vi "Stoppani File Read.vi"(0 "String in":path) -> (3 "run":cluster{"Sampling rate":dbl, "npts":dbl}, 4 "Waveform Graph":T1(graph), 5 "Header Info":T2={"TFRFHeader"={"index"=22, "Xr"=294.1319931548027, "Yr"=349.0, "XActual"=294.1319931548027, "YActual"=349.0}, "Frequency Axis"={"Hz Resolution"=0.67291259765625, "Start Freq"=24.89776611328125, "End Freq"=3500.4913330078125}, "TSingleArray"={"fComplex"=1, "fLength"=5166.0, "a[2]"=0.0, "fConditionCheck"=1.0, "Precision"=0.0, "MtxVecVersion"=420.0, "SizeOf(TSample)"=8.0, "Tag"=0.0, "MtxVecFileCode"=64019.0, "a[9]"=0.0, "a[10]"=0.0}, "caption"="\u0000\u0000\u0000\u0000"}, 6 "Complex FRF":cluster{"t0":dbl, "dt":dbl, "Y":cdb[]})   [LabVIEW 2022 SP3]
panel:
  out "String out":string
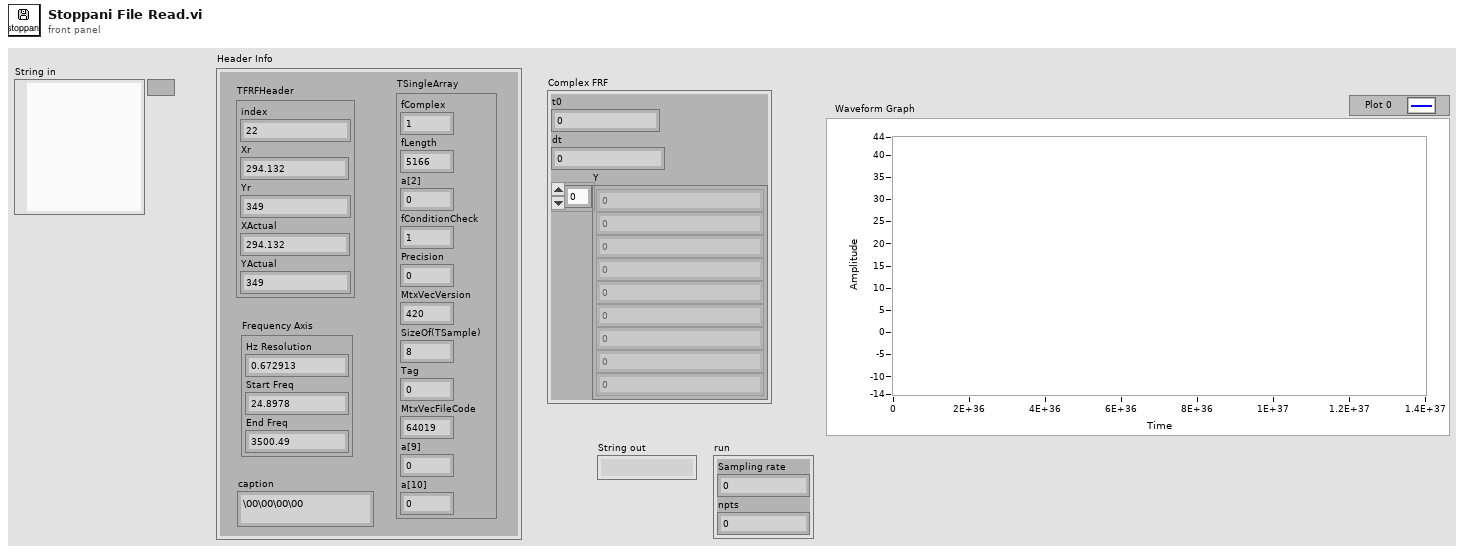
[diagram p1: front panel]
types:
  T1 = cluster{"Start freq":dbl, "Hz resolution":dbl, dbl[]}
  T2 = cluster{"TFRFHeader":cluster{"index":u32, "Xr":dbl, "Yr":dbl, "XActual":dbl, "YActual":dbl}, "Frequency Axis":cluster{"Hz Resolution":dbl, "Start Freq":dbl, "End Freq":dbl}, "TSingleArray":cluster{"fComplex":u32, "fLength":dbl, "a[2]":dbl, "fConditionCheck":dbl, "Precision":dbl, "MtxVecVersion":dbl, "SizeOf(TSample)":dbl, "Tag":dbl, "MtxVecFileCode":dbl, "a[9]":dbl, "a[10]":dbl}, "caption":string}
  T3 = enum16{"big-endian, network order", "native, host order", "little-endian"}
  T4 = cluster{"[0]":dbl, "[1]":dbl, "[2]":dbl, "[3]":dbl, "[4]":dbl}
  T5 = cluster{"[0]":sgl, "[1]":sgl, "[2]":sgl, "[3]":sgl, "[4]":sgl, "[5]":sgl, "[6]":sgl, "[7]":sgl, "[8]":sgl, "[9]":sgl, "[10]":sgl}
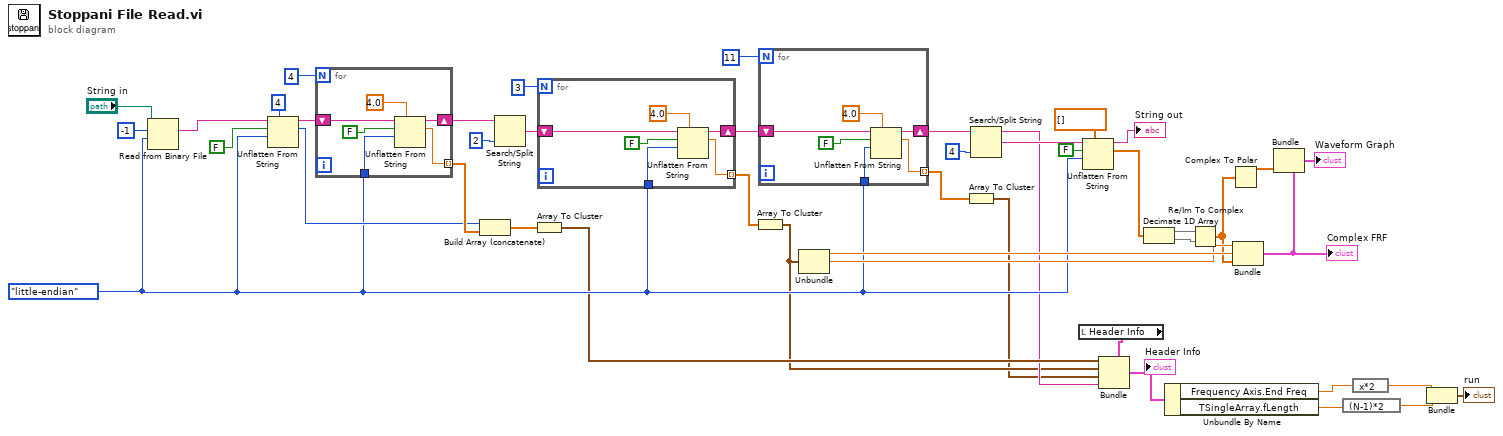
[diagram p0: block diagram]
diagram:
  w16 = T3."little-endian" ("byte order (0:big-endian, network order)")
  n1 = Read from Binary File(9:w16, 10:-1 ("count (1)"), 11:"String in") -> (2:w17:string)  [unwired: 3 in, 3 out]
  n2 = Unflatten From String(type=u32 4 ("count (1)"), binary string=w17, data includes array or string size? (T)=FALSE, byte order (0:big-endian, network order)=w16) -> (rest of the binary string=w31:string, value=w40:u32)  [unwired: 1 in, 1 out]
  n3 = for {
    N: 4 -> [_]
    shift-right: [w48] -> w34
    shift-left: w31 -> [w50]
    tunnel: [w47] -> w42 mode=indexing
    tunnel: w16 -> [w46]
    n4 = Unflatten From String(type=4.0 ("count (1)"), binary string=w50, data includes array or string size? (T)=FALSE, byte order (0:big-endian, network order)=w46) -> (rest of the binary string=w48:string, value=w47:dbl)  [unwired: 1 in, 1 out]
  }
  n5 = Build Array (concatenate)(w40, w42) -> (w43:dbl[])
  n6 = Search/Split String(string=w34, offset (0)=2) -> (match + rest of string=w35:string)  [unwired: 1 in, 2 out]
  n7 = Array To Cluster(array=w43) -> (cluster=w15:T4)
  n8 = for {
    N: 3 -> [_]
    shift-right: [w54] -> w37
    shift-left: w35 -> [w56]
    tunnel: [w53] -> w44 mode=indexing
    tunnel: w16 -> [w52]
    n9 = Unflatten From String(type=4.0 ("count (1)"), binary string=w56, data includes array or string size? (T)=FALSE, byte order (0:big-endian, network order)=w52) -> (rest of the binary string=w54:string, value=w53:dbl)  [unwired: 1 in, 1 out]
  }
  n10 = Array To Cluster(array=w44) -> (cluster=w9:cluster{"[0]":dbl, "[1]":dbl, "[2]":dbl})
  n11 = for {
    N: 11 -> [_]
    shift-right: [w60] -> w39
    shift-left: w37 -> [w62]
    tunnel: [w59] -> w45 mode=indexing
    tunnel: w16 -> [w58]
    n12 = Unflatten From String(type=sgl 4.0 ("count (1)"), binary string=w62, data includes array or string size? (T)=FALSE, byte order (0:big-endian, network order)=w58) -> (rest of the binary string=w60:string, value=w59:sgl)  [unwired: 1 in, 1 out]
  }
  n13 = Unbundle(w9) -> ("[0]"=w28:dbl, "[1]"=w27:dbl)  [unwired: 1 out]
  n14 = Array To Cluster(array=w45) -> (cluster=w6:T5)
  n15 = Search/Split String(string=w39, offset (0)=4) -> (substring before match=w14:string, match + rest of string=w23:string)  [unwired: 1 in, 1 out]
  n16 = local read "Header Info"() -> (w4:T2)
  n17 = Unflatten From String(type=dbl[] [], binary string=w23, data includes array or string size? (T)=FALSE, byte order (0:big-endian, network order)=w16) -> (rest of the binary string=→"String out":string, value=w21:dbl[])  [unwired: 1 in, 1 out]
  n18 = Bundle(cluster=w4, "TFRFHeader"=w15, "Frequency Axis"=w9, "TSingleArray"=w6, "caption"=w14) -> (w5:T2)
  "Header Info" <- w5
  n19 = Decimate 1D Array(w21) -> (w26:dbl[], w25:dbl[])
  n20 = Unbundle By Name(w5) -> ("Frequency Axis.End Freq"=w3:dbl, "TSingleArray.fLength"=w2:dbl)
  n21 = Re/Im To Complex(1:w25, 2:w26) -> (0:w13:cdb[])
  n22 = Complex To Polar(r * e^(i*theta)=w13) -> (r=w11:dbl[])  [unwired: 1 out]
  n23 = Bundle("[1]"=w27, "[0]"=w28, w13) -> (w12:cluster{"[1]":dbl, "[0]":dbl, cdb[]})  [unwired: 1 in]
  "Complex FRF" <- w12
  n24 = Bundle(cluster=w12, w11) -> (→"Waveform Graph":cluster{"[1]":dbl, "[0]":dbl, cdb[]})  [unwired: 2 in]
  n25 = expression code="(N-1)*2"(w2) -> (w1:dbl)
  n26 = expression code="x*2"(w3) -> (w7:dbl)
  n27 = Bundle("End Freq"=w7, "fLength"=w1) -> (→"run":cluster{"End Freq":dbl, "fLength":dbl})  [unwired: 1 in]
